vi "principal.vi"() -> ()   [LabVIEW 2018]
panel:
  in  "stop":bool
  out "6eme note":string
  in  "Moyenne visée":dbl=1.0 min=1.0 max=6.0 step=0.5 format="%#_2g"
  out "Moyenne actuelle":dbl
  out "Notes":dbl[](array[numeric])
  # "Avec"
  # "et je dois faire"
  # "ma moyenne est de"
  # "pour avoir une moyenne de"
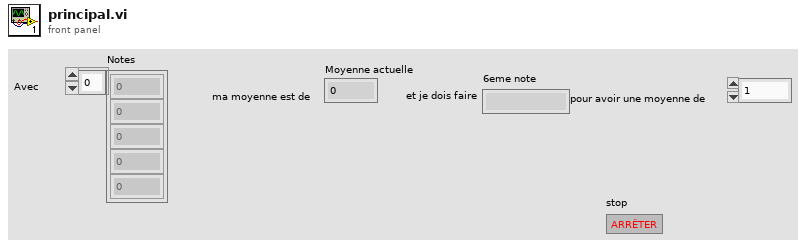
[diagram p1: front panel]
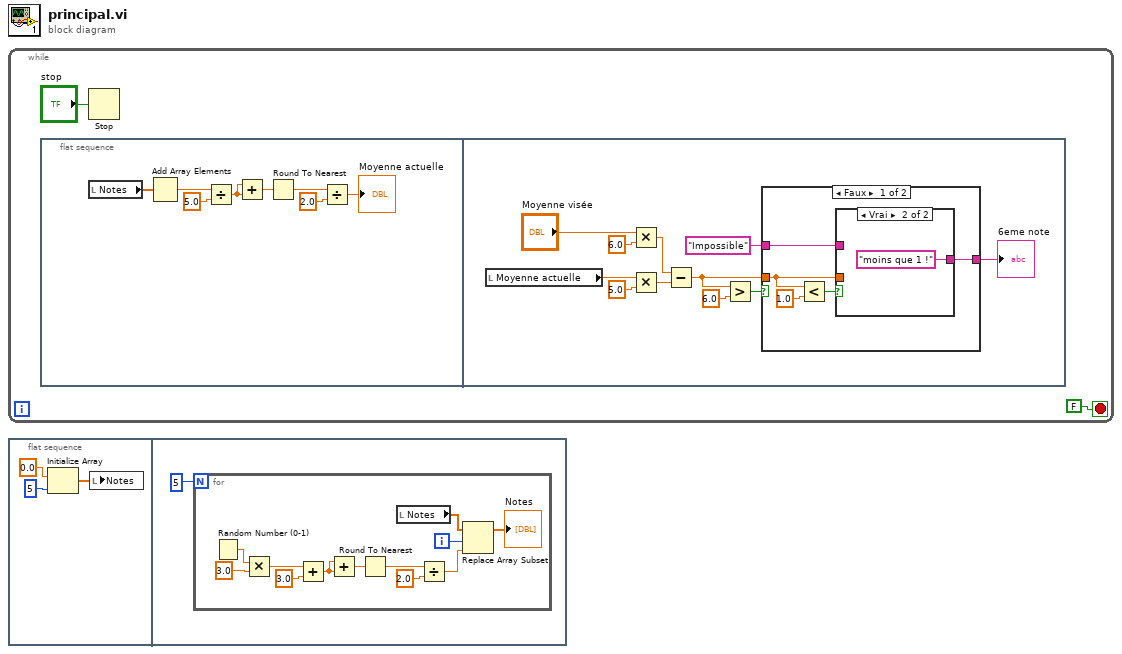
[diagram p0: block diagram]
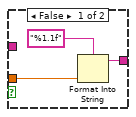
[diagram p2: hidden frame]
diagram:
  n1 = while {
    stop <- FALSE stop-if-true
    n2 = flat-sequence {
      frame #0 {
        n3 = local read "Notes"() -> (w9:dbl[])
        n4 = Add Array Elements(numeric array=w9) -> (sum=w10:dbl)
        n5 = Divide(x=w10, y=5.0 ("x/y")) -> (x/y=w4:dbl)
        n6 = Add(x=w4, y=w4) -> (x+y=w7:dbl)
        n7 = Round To Nearest(number=w7) -> (nearest integer value=w6:dbl)
        n8 = Divide(x=w6, y=2.0) -> (x/y=→"Moyenne actuelle":dbl)
      }
      frame #1 {
        n9 = local read "Moyenne actuelle"() -> (w19:dbl)
        n10 = Multiply(x="Moyenne visée", y=6.0) -> (x*y=w17:dbl)
        n11 = Multiply(x=w19, y=5.0) -> (x*y=w16:dbl)
        n12 = Subtract(x=w17, y=w16) -> (x-y=w13:dbl)
        n13 = Greater?(x=w13, y=6.0) -> (0:w14:bool)
        n14 = case shown="Faux" w14 {
          tunnel: w13 -> [w22 _]
          tunnel: "Impossible" -> [w24 w31]
          tunnel: [w23 w31] -> w11
          frame False {
            n15 = Less?(x=w22, y=1.0) -> (x < y?=w25:bool)
            n16 = case shown="Vrai" w25 {
              tunnel: w24 -> [_ _]
              tunnel: [w29 "moins que 1 !"] -> w23
              tunnel: w22 -> [w27 _]
              frame False {
                n17 = Format Into String(format string="%1.1f" ("chaîne de format"), w27) -> (resulting string=w29:string)  [unwired: 2 in, 1 out]
              }
              frame True {
              }
            }
          }
          frame True {
          }
        }
        "6eme note" <- w11
      }
    }
    n18 = Stop(stop? (T)="stop") -> ()
  }
  n19 = flat-sequence {
    frame #0 {
      n20 = Initialize Array(0.0 ("élément"), 5 ("taille de la dimension")) -> (w34:dbl[])
      n21 = local write "Notes"(w34) -> ()
    }
    frame #1 {
      n22 = for {
        N: 5 -> [_]
        i -> [w37]
        n23 = Random Number (0-1)() -> (number: 0 to 1=w47:dbl)
        n24 = Multiply(x=w47, y=3.0) -> (x*y=w46:dbl)
        n25 = Add(x=w46, y=3.0) -> (x+y=w41:dbl)
        n26 = Add(x=w41, y=w41) -> (x+y=w36:dbl)
        n27 = Round To Nearest(number=w36) -> (nearest integer value=w42:dbl)
        n28 = local read "Notes"() -> (w40:dbl[])
        n29 = Divide(x=w42, y=2.0) -> (x/y=w39:dbl)
        n30 = Replace Array Subset(array=w40, new element=w39, index=w37) -> (→"Notes":dbl[])
      }
    }
  }
